vi "Joystic To Global.vi"   [LabVIEW 2012]
uses:
  Robot Global Data.vi
  <vilib>/Rock Robotics/WPI/Joystick/WPI_JoystickGetSetRefNum.vi
types:
  T1 = typedef "WPI_JoystickDevRef.ctl" = cluster{"Device":T2}
  T2 = typedef "WPI_JoystickDeviceEnum.ctl" = enum16{"USB 1", "USB 2", "USB 3", "USB 4", "Kinect 1", "Kinect 2"}
  T3 = typedef "WPI_JoystickButtonState.ctl" = cluster{"Button 1":bool, "Button 2":bool, "Button 3":bool, "Button 4":bool, "Button 5":bool, "Button 6":bool, "Button 7":bool, "Button 8":bool, "Button 9":bool, "Button 10":bool, "Button 11":bool, "Button 12":bool}
  T4 = cluster{"axis 1 (x)":dbl, "axis 2 (y)":dbl, "axis 3 (throttle)":dbl, "axis 4":dbl, "axis 5":dbl, "axis 6":dbl}
  T5 = cluster{"Driver Station Digital Input (1-8)[0]":bool, "Driver Station Digital Input (1-8)[1]":bool, "Driver Station Digital Input (1-8)[2]":bool, "Driver Station Digital Input (1-8)[3]":bool, "Driver Station Digital Input (1-8)[4]":bool, "Driver Station Digital Input (1-8)[5]":bool, "Driver Station Digital Input (1-8)[6]":bool, "Driver Station Digital Input (1-8)[7]":bool, "Driver Station Digital Input (1-8)[8]":bool}
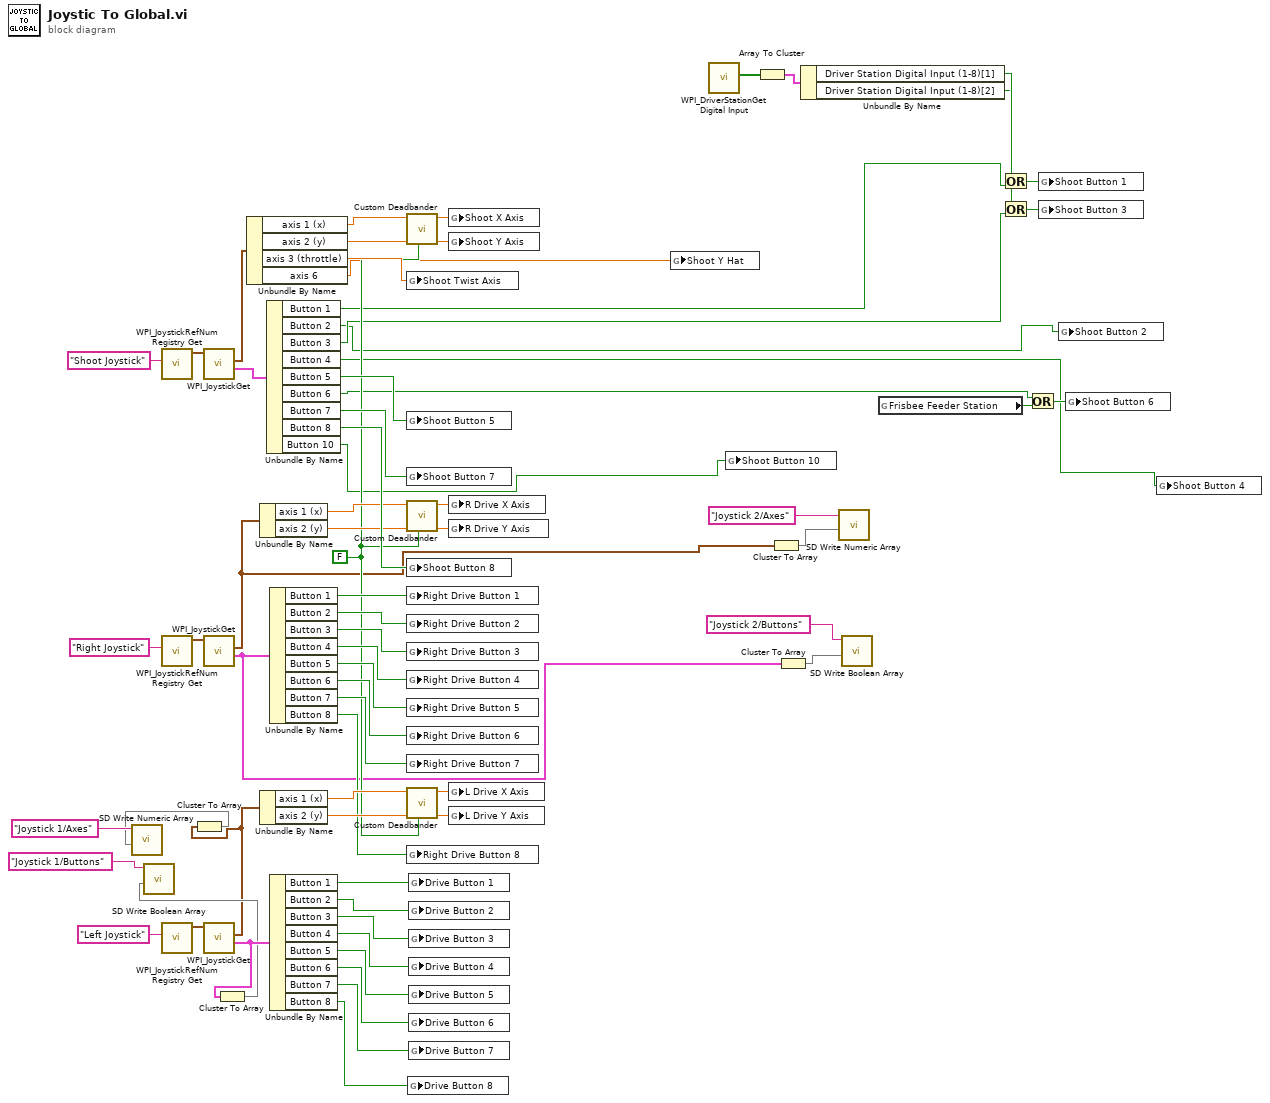
[diagram p0: block diagram]
diagram:
  w28 = FALSE ("Invert (TF)")
  n1 = call <vilib>:"WPI_JoystickRefNum Registry Get.vi"("refnum name"="Shoot Joystick") -> ("JoystickDevRef"=w62:T1)  [unwired: 9 in, 1 out]
  n2 = call <vilib>:"WPI_JoystickRefNum Registry Get.vi"("refnum name"="Right Joystick") -> ("JoystickDevRef"=w33:T1)  [unwired: 9 in, 1 out]
  n3 = call <vilib>:"WPI_JoystickRefNum Registry Get.vi"("refnum name"="Left Joystick") -> ("JoystickDevRef"=w47:T1)  [unwired: 9 in, 1 out]
  n4 = call <vilib>:"WPI_JoystickGet.vi"("JoystickDevRef"=w62) -> ("Buttons"=w65:T3, "Axes"=w64:T4)  [unwired: 4 in, 1 out]
  n5 = call <vilib>:"WPI_JoystickGet.vi"("JoystickDevRef"=w33) -> ("Buttons"=w18:T3, "Axes"=w17:T4)  [unwired: 4 in, 1 out]
  n6 = call <vilib>:"WPI_JoystickGet.vi"("JoystickDevRef"=w47) -> ("Buttons"=w23:T3, "Axes"=w21:T4)  [unwired: 4 in, 1 out]
  n7 = Cluster To Array(cluster=w21) -> (array=w20:dbl[])
  n8 = call <vilib>:"SD Write Numeric Array.vi"("Numeric Array"=w20, "Name"="Joystick 1/Axes") -> ()  [unwired: 8 in, 2 out]
  n9 = Cluster To Array(cluster=w23) -> (array=w22:bool[])
  n10 = call <vilib>:"SD Write Boolean Array.vi"("Boolean Array"=w22, "Name"="Joystick 1/Buttons") -> ()  [unwired: 8 in, 2 out]
  n11 = Unbundle By Name(w64) -> ("axis 1 (x)"=w61:dbl, "axis 2 (y)"=w60:dbl, "axis 3 (throttle)"=w58:dbl, "axis 6"=w14:dbl)
  n12 = Unbundle By Name(w17) -> ("axis 1 (x)"=w32:dbl, "axis 2 (y)"=w31:dbl)
  n13 = Unbundle By Name(w21) -> ("axis 1 (x)"=w46:dbl, "axis 2 (y)"=w45:dbl)
  n14 = Unbundle By Name(w65) -> ("Button 1"=w10:bool, "Button 2"=w5:bool, "Button 3"=w8:bool, "Button 4"=w6:bool, "Button 5"=w66:bool, "Button 6"=w13:bool, "Button 7"=w67:bool, "Button 8"=w68:bool, "Button 10"=w15:bool)
  n15 = Unbundle By Name(w18) -> ("Button 1"=w35:bool, "Button 2"=w36:bool, "Button 3"=w37:bool, "Button 4"=w38:bool, "Button 5"=w39:bool, "Button 6"=w40:bool, "Button 7"=w41:bool, "Button 8"=w42:bool)
  n16 = Unbundle By Name(w23) -> ("Button 1"=w49:bool, "Button 2"=w50:bool, "Button 3"=w51:bool, "Button 4"=w52:bool, "Button 5"=w53:bool, "Button 6"=w54:bool, "Button 7"=w55:bool, "Button 8"=w56:bool)
  n17 = call "Custom Deadbander.vi"("Invert (TF)"=w28, "y"=w60, "x"=w61) -> ("y edited"=w57:dbl, "X edited"=w59:dbl)  [unwired: 7 in]
  n18 = global write "Robot Global Data.vi" "Shoot Twist Axis"(w58) -> ()
  n19 = global write "Robot Global Data.vi" "Shoot Button 5"(w66) -> ()
  n20 = global write "Robot Global Data.vi" "Shoot Button 7"(w67) -> ()
  n21 = call "Custom Deadbander.vi"("Invert (TF)"=w28, "y"=w31, "x"=w32) -> ("y edited"=w29:dbl, "X edited"=w30:dbl)  [unwired: 7 in]
  n22 = global write "Robot Global Data.vi" "Shoot Button 8"(w68) -> ()
  n23 = global write "Robot Global Data.vi" "Right Drive Button 1"(w35) -> ()
  n24 = global write "Robot Global Data.vi" "Right Drive Button 2"(w36) -> ()
  n25 = global write "Robot Global Data.vi" "Right Drive Button 3"(w37) -> ()
  n26 = global write "Robot Global Data.vi" "Right Drive Button 4"(w38) -> ()
  n27 = global write "Robot Global Data.vi" "Right Drive Button 5"(w39) -> ()
  n28 = global write "Robot Global Data.vi" "Right Drive Button 6"(w40) -> ()
  n29 = global write "Robot Global Data.vi" "Right Drive Button 7"(w41) -> ()
  n30 = call "Custom Deadbander.vi"("Invert (TF)"=w28, "y"=w45, "x"=w46) -> ("y edited"=w43:dbl, "X edited"=w44:dbl)  [unwired: 7 in]
  n31 = global write "Robot Global Data.vi" "Right Drive Button 8"(w42) -> ()
  n32 = global write "Robot Global Data.vi" "Drive Button 8"(w56) -> ()
  n33 = global write "Robot Global Data.vi" "Drive Button 1"(w49) -> ()
  n34 = global write "Robot Global Data.vi" "Drive Button 2"(w50) -> ()
  n35 = global write "Robot Global Data.vi" "Drive Button 3"(w51) -> ()
  n36 = global write "Robot Global Data.vi" "Drive Button 4"(w52) -> ()
  n37 = global write "Robot Global Data.vi" "Drive Button 5"(w53) -> ()
  n38 = global write "Robot Global Data.vi" "Drive Button 6"(w54) -> ()
  n39 = global write "Robot Global Data.vi" "Drive Button 7"(w55) -> ()
  n40 = global write "Robot Global Data.vi" "Shoot X Axis"(w59) -> ()
  n41 = global write "Robot Global Data.vi" "Shoot Y Axis"(w57) -> ()
  n42 = global write "Robot Global Data.vi" "R Drive X Axis"(w30) -> ()
  n43 = global write "Robot Global Data.vi" "R Drive Y Axis"(w29) -> ()
  n44 = global write "Robot Global Data.vi" "L Drive X Axis"(w44) -> ()
  n45 = global write "Robot Global Data.vi" "L Drive Y Axis"(w43) -> ()
  n46 = global write "Robot Global Data.vi" "Shoot Y Hat"(w14) -> ()
  n47 = call <vilib>:"WPI_DriverStationGet Digital Input.vi"() -> ("Driver Station Digital Input (1-8)"=w4:bool[])  [unwired: 11 in]
  n48 = global write "Robot Global Data.vi" "Shoot Button 10"(w15) -> ()
  n49 = Array To Cluster(array=w4) -> (cluster=w3:T5)
  n50 = Cluster To Array(cluster=w17) -> (array=w16:dbl[])
  n51 = Cluster To Array(cluster=w18) -> (array=w19:bool[])
  n52 = Unbundle By Name(w3) -> ("Driver Station Digital Input (1-8)[1]"=w2:bool, "Driver Station Digital Input (1-8)[2]"=w1:bool)
  n53 = call <vilib>:"SD Write Numeric Array.vi"("Numeric Array"=w16, "Name"="Joystick 2/Axes") -> ()  [unwired: 8 in, 2 out]
  n54 = call <vilib>:"SD Write Boolean Array.vi"("Boolean Array"=w19, "Name"="Joystick 2/Buttons") -> ()  [unwired: 8 in, 2 out]
  n55 = global read "Robot Global Data.vi" "Frisbee Feeder Station"() -> (w12:bool)
  n56 = Or(x=w2, y=w10) -> (x .or. y?=w9:bool)
  n57 = Or(x=w1, y=w8) -> (x .or. y?=w7:bool)
  n58 = Or(x=w13, y=w12) -> (x .or. y?=w11:bool)
  n59 = global write "Robot Global Data.vi" "Shoot Button 1"(w9) -> ()
  n60 = global write "Robot Global Data.vi" "Shoot Button 3"(w7) -> ()
  n61 = global write "Robot Global Data.vi" "Shoot Button 2"(w5) -> ()
  n62 = global write "Robot Global Data.vi" "Shoot Button 6"(w11) -> ()
  n63 = global write "Robot Global Data.vi" "Shoot Button 4"(w6) -> ()
